vi "DFD Load NStage MRate Filter from File.vi"(8 "error in (no error)":errorcluster, 10 "file path in":path) -> (0 "error out":errorcluster, 2 "file path out":path, 3 "multirate filters out":T1[](array[typedef]) {"mMRate_SumWl" min=1 max=32 step=1; "mMRate_InputIwl" min=1 max=32 step=1; "mMRate_GainWl" min=1 max=32 step=1; "mMRate_OutputWl" min=1 max=32 step=1; "mMRate_InputWl" min=1 max=32 step=1; "mMRate_CoefWl" min=1 max=32 step=1; "mMRate_Mode" items=["Default"=-1, "No Rate Change"=0, "Interpolation"=1, "Decimation"=2, "Interpolated"=3, "Rational"=4]})   [LabVIEW 2017, in "NI_DigFilterLicensed.lvlib"]
doc: "Retrieves a filter or a filter bank from a file. You must manually select the polymorphic instance you want to use."
uses:
  <vilib>/addons/Digital Filter Design/NI_DigFilterLicensed.lvlib
  <vilib>/addons/Digital Filter Design/_Objects.llb/DFD Multirate Filter Obj.ctl
  <vilib>/addons/Digital Filter Design/_Objects.llb/DFD Multirate Mode.ctl
  <vilib>/addons/Digital Filter Design/_Objects.llb/DFD Coef Norm Type.ctl
  <vilib>/addons/Digital Filter Design/_Objects.llb/DFD Round-off Mode.ctl
  <vilib>/addons/Digital Filter Design/_Objects.llb/DFD FXP MRate Multiply Mode.ctl
  <vilib>/addons/Digital Filter Design/_Misc.llb/dfd_Error Handlers (Single).vi
panel:
  in  "multirate filter":T1={"mMRate_Structure"=enum."CIC", "mMRate_Mode"=0, "mMRate_Factor"=1, "mMRate_FIRParams"={"mMRate_FIR_H"=[], "mMRate_FIR_IsNyquist?"=FALSE, "mMRate_FIR_IsSymmetric?"=FALSE}, "mMRate_CICParams"={"mMRate_CIC_#Stage"=2, "mMRate_CIC_Lag"=1, "mMRate_CIC_Type"=enum."Lowpass"}, "mMRate_Order"=1, "mMRate_Version"="1.0", "mMRate_Comments"="1.0", "mMRate_RationalFactor"={"mMRate_L"=-1, "mMRate_M"=-1}, "mMRate_Fs"=0.0, "mMRate_Quantized?"=FALSE, "mMRate_QFilterGain"=1.0, "mMRate_CoefWl"=16, "mMRate_Scaling"={"mMRate_ScaleByPowerOf2?"=FALSE, "mMRate_ScaleType"=enum."Time Domain 1-Norm"}, "mMRate_InputWl"=0, "mMRate_OutputWl"=0, "mMRate_OutputMode"=enum."Nearest", "mMRate_MultMode"=enum."Full", "mMRate_BitPruning"=FALSE, "mMRate_GainWl"=16, "mMRate_OutputFwl"=0, "mMRate_SumIwl"=0, "mMRate_InputIwl "=16, "mMRate_SumWl"=32, "mMRate_CoefIwl"=0} {"mMRate_SumWl" min=1 max=32 step=1; "mMRate_InputIwl" min=1 max=32 step=1; "mMRate_GainWl" min=1 max=32 step=1; "mMRate_OutputWl" min=1 max=32 step=1; "mMRate_InputWl" min=1 max=32 step=1; "mMRate_CoefWl" min=1 max=32 step=1; "mMRate_Mode" items=["Default"=-1, "No Rate Change"=0, "Interpolation"=1, "Decimation"=2, "Interpolated"=3, "Rational"=4]}
  in  "multirate filters in":T1[](array[typedef]) {"mMRate_SumWl" min=1 max=32 step=1; "mMRate_InputIwl" min=1 max=32 step=1; "mMRate_GainWl" min=1 max=32 step=1; "mMRate_OutputWl" min=1 max=32 step=1; "mMRate_InputWl" min=1 max=32 step=1; "mMRate_CoefWl" min=1 max=32 step=1; "mMRate_Mode" items=["Default"=-1, "No Rate Change"=0, "Interpolation"=1, "Decimation"=2, "Interpolated"=3, "Rational"=4]}
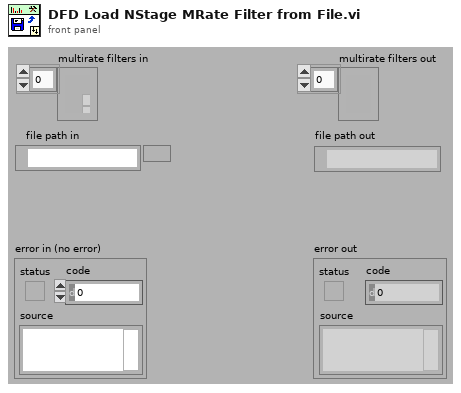
[diagram p1: front panel]
types:
  T1 = typedef "NI_DigFilterLicensed.lvlib/DFD Multirate Filter Obj.ctl" = cluster{"mMRate_Structure":enum16{"CIC", "FIR", "IIR", "Lattice"}, "mMRate_Mode":T2, "mMRate_Factor":i32, "mMRate_FIRParams":cluster{"mMRate_FIR_H":dbl[], "mMRate_FIR_IsNyquist?":bool, "mMRate_FIR_IsSymmetric?":bool}, "mMRate_CICParams":cluster{"mMRate_CIC_#Stage":i32, "mMRate_CIC_Lag":i32, "mMRate_CIC_Type":enum16{"Lowpass", "Highpass"}}, "mMRate_Order":i32, "mMRate_Version":string, "mMRate_Comments":string, "mMRate_RationalFactor":cluster{"mMRate_L":i32, "mMRate_M":i32}, "mMRate_Fs":dbl, "mMRate_Quantized?":bool, "mMRate_QFilterGain":dbl, "mMRate_CoefWl":i16, "mMRate_Scaling":cluster{"mMRate_ScaleByPowerOf2?":bool, "mMRate_ScaleType":T3}, "mMRate_InputWl":i16, "mMRate_OutputWl":i16, "mMRate_OutputMode":T4, "mMRate_MultMode":T5, "mMRate_BitPruning":bool, "mMRate_GainWl":i16, "mMRate_OutputFwl":i16, "mMRate_SumIwl":i16, "mMRate_InputIwl ":i16, "mMRate_SumWl":i16, "mMRate_CoefIwl":i16}
  T2 = typedef "NI_DigFilterLicensed.lvlib/DFD Multirate Mode.ctl" = i16
  T3 = typedef "NI_DigFilterLicensed.lvlib/DFD Coef Norm Type.ctl" = enum16{"No Norm", "Time Domain 1-Norm", "Time Domain 2-Norm", "Time Domain Inf-Norm"}
  T4 = typedef "NI_DigFilterLicensed.lvlib/DFD Round-off Mode.ctl" = enum16{"Nearest", "Truncation"}
  T5 = typedef "NI_DigFilterLicensed.lvlib/DFD FXP MRate Multiply Mode.ctl" = enum16{"Truncated", "Full"}
  T6 = enum16{"open", "open or create", "create or replace", "create", "open (read only)"}
  T7 = cluster{"mMRate_Structure":enum16{"CIC", "FIR", "IIR", "Lattice"}, "mMRate_Mode":T2, "mMRate_Factor":i32, "mMRate_FIRParams":cluster{"mMRate_FIR_H":dbl[], "mMRate_FIR_IsNyquist?":bool, "mMRate_FIR_IsSymmetric?":bool}, "mMRate_CICParams":cluster{"mMRate_CIC_#Stage":i32, "mMRate_CIC_Lag":i32, "mMRate_CIC_Type":enum16{"Lowpass", "Highpass"}}, "mMRate_Order":i32, "mMRate_Version":string, "mMRate_Comments":string}
  T8 = cluster{"mMRate_Structure":enum16{"CIC", "FIR", "IIR", "Lattice"}, "mMRate_Mode":T2, "mMRate_Factor":i32, "mMRate_FIRParams":cluster{"mMRate_FIR_H":dbl[], "mMRate_FIR_IsNyquist?":bool, "mMRate_FIR_IsSymmetric?":bool}, "mMRate_CICParams":cluster{"mMRate_CIC_#Stage":i32, "mMRate_CIC_Lag":i32, "mMRate_CIC_Type":enum16{"Lowpass", "Highpass"}}, "mMRate_Order":i32, "mMRate_Version":string, "mMRate_Comments":string, "mMRate_RationalFactor":cluster{"mMRate_L":i32, "mMRate_M":i32}, "mMRate_Fs":dbl, "mMRate_Quantized?":bool, "mMRate_QFilterGain":dbl, "mMRate_CoefWl":i16, "mMRate_Scaling":cluster{"mMRate_ScaleByPowerOf2?":bool, "mMRate_ScaleType":T3}, "mMRate_InputWl":i16, "mMRate_OutputWl":i16, "mMRate_OutputMode":T4, "mMRate_MultMode":T5, "mMRate_BitPruning":bool, "mMRate_GainWl":i16, "mMRate_OutputFwl":i16, "mMRate_SumIwl":i16}
  T9 = cluster{"mMRate_Structure":enum16{"CIC", "FIR", "IIR", "Lattice"}, "mMRate_Mode":T2, "mMRate_Factor":i32, "mMRate_FIRParams":cluster{"mMRate_FIR_H":dbl[], "mMRate_FIR_IsNyquist?":bool, "mMRate_FIR_IsSymmetric?":bool}, "mMRate_CICParams":cluster{"mMRate_CIC_#Stage":i32, "mMRate_CIC_Lag":i32, "mMRate_CIC_Type":enum16{"Lowpass", "Highpass"}}, "mMRate_Order":i32, "mMRate_Version":string, "mMRate_Comments":string}[]
  T10 = cluster{"mMRate_Structure":enum16{"CIC", "FIR", "IIR", "Lattice"}, "mMRate_Mode":T2, "mMRate_Factor":i32, "mMRate_FIRParams":cluster{"mMRate_FIR_H":dbl[], "mMRate_FIR_IsNyquist?":bool, "mMRate_FIR_IsSymmetric?":bool}, "mMRate_CICParams":cluster{"mMRate_CIC_#Stage":i32, "mMRate_CIC_Lag":i32, "mMRate_CIC_Type":enum16{"Lowpass", "Highpass"}}, "mMRate_Order":i32, "mMRate_Version":string, "mMRate_Comments":string, "mMRate_RationalFactor":cluster{"mMRate_L":i32, "mMRate_M":i32}, "mMRate_Fs":dbl, "mMRate_Quantized?":bool, "mMRate_QFilterGain":dbl, "mMRate_CoefWl":i16, "mMRate_Scaling":cluster{"mMRate_ScaleByPowerOf2?":bool, "mMRate_ScaleType":T3}, "mMRate_InputWl":i16, "mMRate_OutputWl":i16, "mMRate_OutputMode":T4, "mMRate_MultMode":T5, "mMRate_BitPruning":bool, "mMRate_GainWl":i16, "mMRate_OutputFwl":i16, "mMRate_SumIwl":i16}[]
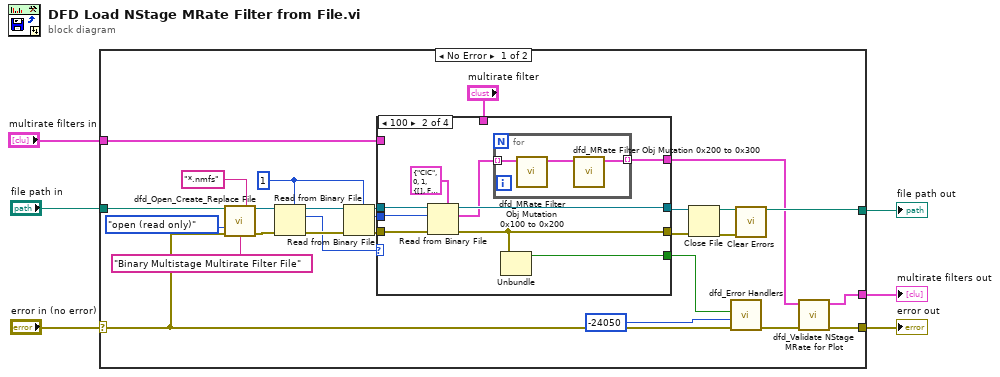
[diagram p0: block diagram]
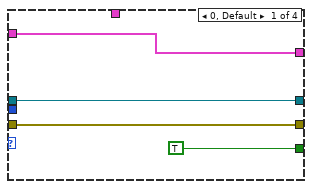
[diagram p2: hidden frame]
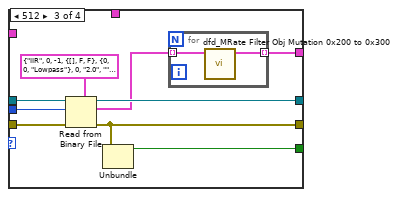
[diagram p3: hidden frame]
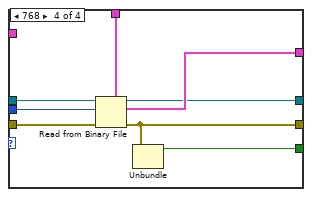
[diagram p4: hidden frame]
diagram:
  n1 = case shown="No Error" "error in (no error)" {
    selector: "error in (no error)" -> [w27 w70]
    tunnel: [w9 w70] -> w5
    tunnel: "file path in" -> [w20 w68]
    tunnel: "multirate filters in" -> [w16 w69]
    tunnel: [w7 w69] -> w1
    tunnel: [w29 w68] -> w3
    frame No Error {
      w21 = 1 ("count")
      n2 = call <vilib>:"dfd_Open_Create_Replace File.vi"("file path"=w20, "pattern"="*.nmfs", "function (open:0)"=T6."open (read only)", "error in (no error)"=w27, "pattern label"="Binary Multistage Multirate Filter File") -> ("refnum"=w31:refnum<file>, "error out"=w30:errorcluster)  [unwired: 3 in, 6 out]
      n3 = Read from Binary File(5:w21, 8:w30, 11:w31) -> (0:w22:errorcluster, 2:w14:i32, 3:w23:refnum<file>)  [unwired: 4 out]
      n4 = Read from Binary File(5:w21, 8:w22, 11:w23) -> (0:w17:errorcluster, 2:w13:i32, 3:w18:refnum<file>)  [unwired: 1 in, 3 out]
      n5 = case shown="100" w14 {
        tunnel: w16 -> [w33 _ _ _]
        tunnel: [w33 w37 w49 w63] -> w8
        tunnel: w18 -> [w35 w41 w57 w65]
        tunnel: w17 -> [w34 w45 w56 w64]
        tunnel: [w35 w44 w55 w61] -> w12
        tunnel: [w34 w43 w54 w62] -> w11
        tunnel: [TRUE ("status") w42 w53 w60] -> w19
        tunnel: "multirate filter" -> [_ _ _ w67]
        tunnel: w13 -> [_ w38 w52 w66]
        frame 0, Default {
        }
        frame 256 {
          n6 = Read from Binary File(5:T7 {"mMRate_Structure"=enum."CIC", "mMRate_Mode"=0, "mMRate_Factor"=1, "mMRate_FIRParams"={"mMRate_FIR_H"=[], "mMRate_FIR_IsNyquist?"=FALSE, "mMRate_FIR_IsSymmetric?"=FALSE}, "mMRate_CICParams"={"mMRate_CIC_#Stage"=0, "mMRate_CIC_Lag"=1, "mMRate_CIC_Type"=enum."Lowpass"}, "mMRate_Order"=0, "mMRate_Version"="1.0", "mMRate_Comments"=""} ("multirate filter in"), 8:w45, 10:w38, 11:w41) -> (0:w43:errorcluster, 2:w40:T9, 3:w44:refnum<file>)  [unwired: 1 in, 2 out]
          n7 = for {
            tunnel: w40 -> [w48] mode=indexing
            tunnel: [w46] -> w37 mode=indexing
            n8 = call <vilib>:"dfd_MRate Filter Obj Mutation 0x100 to 0x200.vi"("multirate filter in (0x100)"=w48) -> ("multirate filter out (0x200)"=w47:T8)  [unwired: 10 out]
            n9 = call <vilib>:"dfd_MRate Filter Obj Mutation 0x200 to 0x300.vi"("multirate filter 200"=w47) -> ("multirate filter out"=w46:T1)  [unwired: 1 in, 9 out]
          }
          n10 = Unbundle(w43) -> ("status"=w42:bool)  [unwired: 2 out]
        }
        frame 512 {
          n11 = Read from Binary File(5:T8 {"mMRate_Structure"=enum."IIR", "mMRate_Mode"=0, "mMRate_Factor"=-1, "mMRate_FIRParams"={"mMRate_FIR_H"=[], "mMRate_FIR_IsNyquist?"=FALSE, "mMRate_FIR_IsSymmetric?"=FALSE}, "mMRate_CICParams"={"mMRate_CIC_#Stage"=0, "mMRate_CIC_Lag"=0, "mMRate_CIC_Type"=enum."Lowpass"}, "mMRate_Order"=0, "mMRate_Version"="2.0", "mMRate_Comments"="", "mMRate_RationalFactor"={"mMRate_L"=-1, "mMRate_M"=-1}, "mMRate_Fs"=1.0, "mMRate_Quantized?"=FALSE, "mMRate_QFilterGain"=1.0, "mMRate_CoefWl"=16, "mMRate_Scaling"={"mMRate_ScaleByPowerOf2?"=FALSE, "mMRate_ScaleType"=enum."No Norm"}, "mMRate_InputWl"=16, "mMRate_OutputWl"=16, "mMRate_OutputMode"=enum."Truncation", "mMRate_MultMode"=enum."Truncated", "mMRate_BitPruning"=FALSE, "mMRate_GainWl"=16, "mMRate_OutputFwl"=0, "mMRate_SumIwl"=0} ("multirate filter in"), 8:w56, 10:w52, 11:w57) -> (0:w54:errorcluster, 2:w50:T10, 3:w55:refnum<file>)  [unwired: 3 out]
          n12 = Unbundle(w54) -> ("status"=w53:bool)  [unwired: 2 out]
          n13 = for {
            tunnel: w50 -> [w59] mode=indexing
            tunnel: [w58] -> w49 mode=indexing
            n14 = call <vilib>:"dfd_MRate Filter Obj Mutation 0x200 to 0x300.vi"("multirate filter 200"=w59) -> ("multirate filter out"=w58:T1)  [unwired: 1 in, 9 out]
          }
        }
        frame 768 {
          n15 = Read from Binary File(5:w67, 8:w64, 10:w66, 11:w65) -> (0:w62:errorcluster, 2:w63:T1[], 3:w61:refnum<file>)  [unwired: 3 out]
          n16 = Unbundle(w62) -> ("status"=w60:bool)  [unwired: 2 out]
        }
      }
      n17 = Close File(refnum=w12, error in=w11) -> (path=w29:path, error out=w26:errorcluster)
      n18 = call-poly <vilib>:"dfd_Error Handlers.vi"("error in (no error)"=w27, "error code"=-24050 ("ERR_FAIL_TO_LOAD"), "condition failed?"=w19) -> ("error out"=w10:errorcluster)  [unwired: 8 out]
      n19 = call <vilib>:"Clear Errors.vi"("error in (no error)"=w26) -> ()  [unwired: 1 in, 6 out]
      n20 = call <vilib>:"dfd_Validate NStage MRate for Plot.vi"("error in (no error)"=w10, "multirate filters in"=w8) -> ("error out"=w9:errorcluster, "multirate filters out"=w7:T1[])  [unwired: 8 out]
    }
    frame Error {
    }
  }
  "error out" <- w5
  "file path out" <- w3
  "multirate filters out" <- w1
